vi "GUNSC_LibSetArrangeSections_left.vi"(8 "error in (no error)":errorcluster, 9 "how":string, 11 "Database RefNum out":T1) -> (0 "error out":errorcluster, 1 "response":string, 2 "return value":i32)   [LabVIEW 2016]
uses:
  DBSHAND/private/vis/DatabaseHand_RefNum.ctl
  DBSHAND/private/vis/DatabaseHand_Element_Set(string).vi
  public/c/lib/libunsc.so
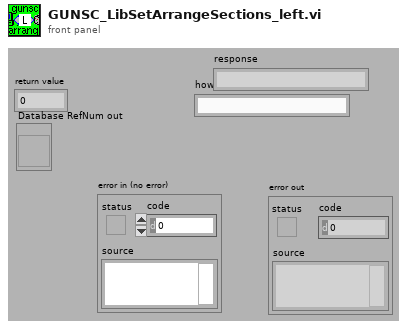
[diagram p1: front panel]
types:
  T1 = typedef "DatabaseHand_RefNum.ctl" = refnum<vi>
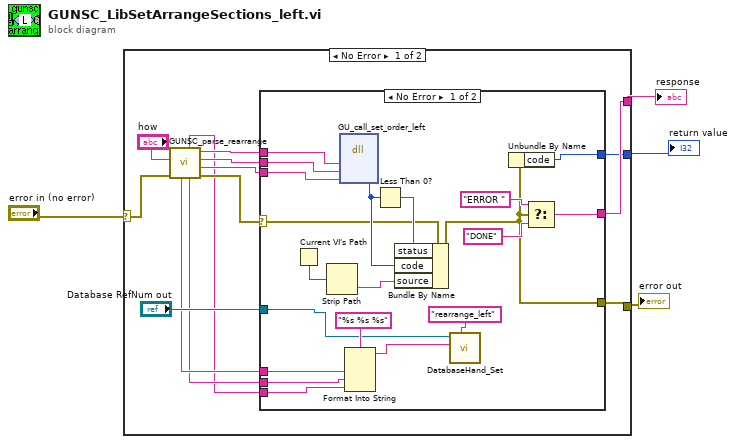
[diagram p0: block diagram]
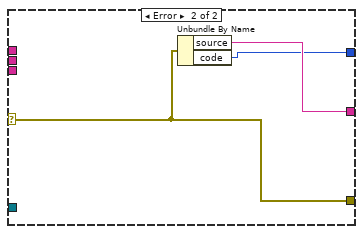
[diagram p2: hidden frame]
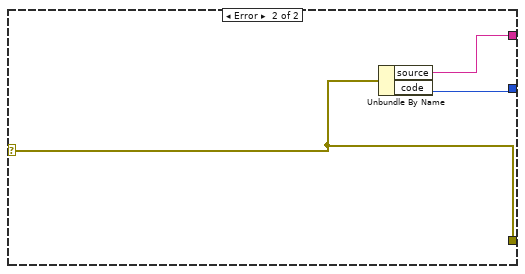
[diagram p3: hidden frame]
diagram:
  n1 = case shown="No Error" "error in (no error)" {
    selector: "error in (no error)" -> [w13 w43]
    tunnel: [w16 w42] -> w4
    tunnel: [w15 w43] -> w2
    tunnel: [w17 w41] -> w1
    frame No Error {
      n2 = call "GUNSC_parse_rearrange.vi"("error in (no error)"=w13, "arguments"="how") -> ("error out"=w12:errorcluster, "func 3"=w9:string, "func 2"=w10:string, "func1"=w11:string, "name2"=w6:string, "name3"=w5:string, "name1"=w7:string)  [unwired: 1 in, 2 out]
      n3 = case shown="No Error" w12 {
        selector: w12 -> [w28 w40]
        tunnel: [w35 w39] -> w17
        tunnel: [w34 w38] -> w16
        tunnel: [w33 w40] -> w15
        tunnel: w11 -> [w24 _]
        tunnel: w10 -> [w23 _]
        tunnel: w9 -> [w22 _]
        tunnel: "Database RefNum out" -> [w21 _]
        tunnel: w7 -> [w20 _]
        tunnel: w6 -> [w19 _]
        tunnel: w5 -> [w18 _]
        frame No Error {
          n4 = Current VI's Path() -> (path=w31:path)
          n5 = Strip Path(path=w31) -> (name=w30:string)  [unwired: 1 out]
          n6 = dll-call lib="home/simager/panview/PAN/Modules/GUNSC/public/c/lib/libunsc.so" fn="GU_call_set_order_left"("left1"=w24, "left2"=w23, "left3"=w22) -> ("return type"=w32:i32)  [unwired: 6 in, 2 out]
          n7 = Format Into String(format string="%s %s %s", w20, w19, w18) -> (resulting string=w25:string)  [unwired: 2 in, 1 out]
          n8 = Less Than 0?(x=w32) -> (x < 0?=w29:bool)
          n9 = Bundle By Name(cluster=w28, "status"=w29, "code"=w32, "source"=w30) -> (w33:errorcluster)
          n10 = call-poly "DatabaseHand_Set.vi"("name"="rearrange_left", "value"=w25, "Database RefNum in"=w21) -> ()  [unwired: 5 in, 4 out]
          n11 = Unbundle By Name(w33) -> ("code"=w34:i32)
          n12 = Select(t="ERROR ", s=w33, f="DONE" ("source")) -> (s? t:f=w35:string)
        }
        frame Error {
          n13 = Unbundle By Name(w40) -> ("source"=w39:string, "code"=w38:i32)
        }
      }
    }
    frame Error {
      n14 = Unbundle By Name(w43) -> ("source"=w41:string, "code"=w42:i32)
    }
  }
  "return value" <- w4
  "error out" <- w2
  "response" <- w1
